vi "Append Formatted Text.vi"(8 "error in (no error)":errorcluster, 9 "Heading Level (-1)":i32(ring)=-1 items=["Title"=0, "H1"=1, "H2"=2, "H3"=3, "H4"=4, "Paragraph"=-1], 10 "Heading Text":string, 11 "Document in":refnum<class "Document.lvclass">) -> (0 "error out":errorcluster, 3 "Document out":refnum<class "Document.lvclass">)   [LabVIEW 2017, in "LabVIEW NPOI.lvlib" / "Document.lvclass"]
doc: "Appends <B>Heading Text</B> to the <B>Document</B> formatted based on the givent <B>Heading Level</B>."
uses:
  Document.lvclass
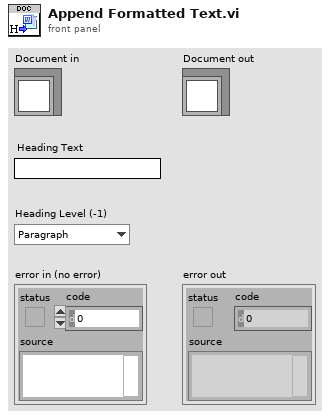
[diagram p1: front panel]
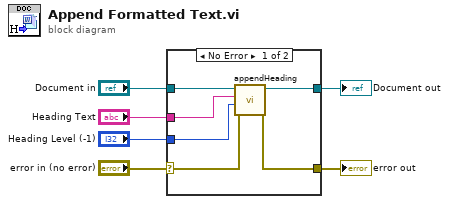
[diagram p0: block diagram]
diagram:
  n1 = case shown="No Error" "error in (no error)" {
    selector: "error in (no error)" -> [w10 w14]
    tunnel: [w9 w14] -> w5
    tunnel: [w11 w13] -> w3
    tunnel: "Document in" -> [w12 w13]
    tunnel: "Heading Text" -> [w8 _]
    tunnel: "Heading Level (-1)" -> [w7 _]
    frame No Error {
      n2 = call-dynamic "appendHeading.vi"("error in (no error)"=w10, "Heading Level (-1)"=w7, "Heading Text"=w8, "Document in"=w12) -> ("error out"=w9:errorcluster, "Document out"=w11:refnum<class "Document.lvclass">)  [unwired: 6 in]
    }
    frame Error {
    }
  }
  "error out" <- w5
  "Document out" <- w3
